vi "JTAG F-RAM Special Config.vi"() -> ()   [LabVIEW 2009]
panel:
  in  "Front Panel":T1 {"Working..." scale=0.0..1.0; "0x7FC5 - STIM ASIC REV" format="%02x"; "FRAM STIM DATA"."Data" format="%02x"; "FRAM STIM DATA"."Address" format="%04x"; "MICS_TRIMS (0x7FF0-7FFF" format="%02x"; "PWR_TRIMS (0x7FD0-7FDF" format="%02x"; "STIM_TRIMS (0x7FE0-7FEF" format="%02x"}
  # "0x7FC0 - STARTUP"
  # "0x7FC4 - SPCL TEST"
  # "0x7FC1 - STIM"
  # "0x7FC2 - PWR"
  # "0x7FC3 - MICS"
  # "BG_TRIM"
  # "PWR_TRIM0"
  # "TX RF Power"
  # "CG_TRIM"
  # "PWR_TRIM1"
  # "TxPort_TxMode"
  # "PGO_TRIM"
  # "PWR_TRIM2"
  # "TxPort_RxMode"
  # "CM_TRIM"
  # "PWR_TRIM3"
  # "RxPort_TxMode"
  # "<Reserved>"
  # "PWR_TRIM4"
  # "RxPort_RxMode"
  # "<Reserved>"
  # "PWR_TRIM5"
  # "Ant_Match1"
  # "<Reserved>"
  # "PWR_TRIM6"
  # "Ant_Match2"
  # "<Reserved>"
  # "PWR_TRIM7"
  # "MICS Channel"
  # "<Reserved>"
  # "PWR_TRIM8"
  # "TX Modulation"
  # "<Reserved>"
  # "PWR_TRIM9"
  # "<Reserved>"
  # "<Reserved>"
  # "PWR_TRIM10"
  # "<Reserved>"
  # "<Reserved>"
  # "<Reserved>"
  # "<Reserved>"
  # "<Reserved>"
  # "<Reserved>"
  # "<Reserved>"
  # "<Reserved>"
  # "<Reserved>"
  # "<Reserved>"
  # "<Reserved>"
  # "<Reserved>"
  # "mac_calselect1"
  # "<Reserved>"
  # "<Reserved>"
  # "mac_calselect2"
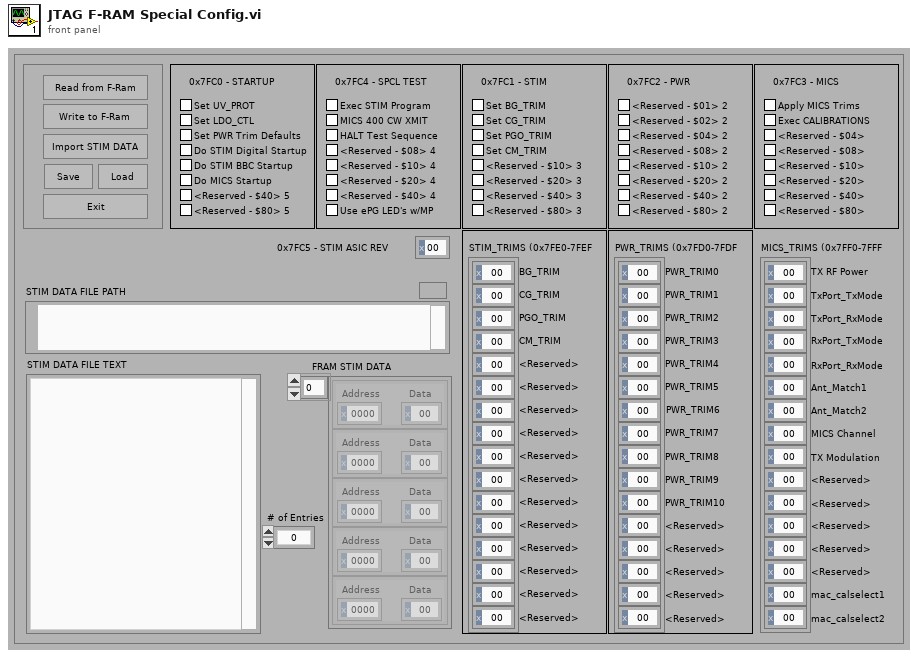
[diagram p1: front panel]
types:
  T1 = cluster{"FRAM STIM DATA":cluster{"Address":u16, "Data":u8}[], "MICS_TRIMS (0x7FF0-7FFF":u8[], "<Reserved - $80>":bool, "<Reserved - $40>":bool, "<Reserved - $20>":bool, "<Reserved - $10>":bool, "<Reserved - $08>":bool, "<Reserved - $04>":bool, "Exec CALIBRATIONS":bool, "Apply MICS Trims":bool, "PWR_TRIMS (0x7FD0-7FDF":u8[], "STIM_TRIMS (0x7FE0-7FEF":u8[], "<Reserved - $80> 2":bool, "<Reserved - $40> 2":bool, "<Reserved - $20> 2":bool, "<Reserved - $10> 2":bool, "<Reserved - $08> 2":bool, "<Reserved - $04> 2":bool, "<Reserved - $02> 2":bool, "<Reserved - $01> 2":bool, "<Reserved - $80> 3":bool, "<Reserved - $40> 3":bool, "<Reserved - $20> 3":bool, "<Reserved - $10> 3":bool, "Set CM_TRIM":bool, "Set PGO_TRIM":bool, "Set CG_TRIM":bool, "Set BG_TRIM":bool, "Use ePG LED's w/MP":bool, "<Reserved - $40> 4":bool, "<Reserved - $20> 4":bool, "<Reserved - $10> 4":bool, "<Reserved - $08> 4":bool, "HALT Test Sequence":bool, "MICS 400 CW XMIT":bool, "Exec STIM Program":bool, "<Reserved - $80> 5":bool, "<Reserved - $40> 5":bool, "Do MICS Startup":bool, "Do STIM BBC Startup":bool, "Do STIM Digital Startup":bool, "Set PWR Trim Defaults":bool, "Set LDO_CTL":bool, "Set UV_PROT":bool, "STIM DATA FILE PATH":path, "STIM DATA FILE TEXT":string, "# of Entries":u16, "User Controls":cluster{"Exit":bool, "Import Stim Prog":bool, "Write to F-Ram":bool, "Read from F-Ram":bool, "Save":bool, "Load":bool}, "0x7FC5 - STIM ASIC REV":u8, "Working...":dbl}
  T2 = cluster{"STIM PROGRAM FRAM DATA":cluster{"Address":u16, "Data":u8}[], "MICS_TRIMS (0x7FF0-7FFF":u8[], "<Reserved - $80>":bool, "<Reserved - $40>":bool, "<Reserved - $20>":bool, "<Reserved - $10>":bool, "<Reserved - $08>":bool, "<Reserved - $04>":bool, "<Reserved - $02>":bool, "<Reserved - $01>":bool, "PWR_TRIMS (0x7FD0-7FDF":u8[], "STIM_TRIMS (0x7FE0-7FEF":u8[], "<Reserved - $80> 2":bool, "<Reserved - $40> 2":bool, "<Reserved - $20> 2":bool, "<Reserved - $10> 2":bool, "<Reserved - $08> 2":bool, "<Reserved - $04> 2":bool, "<Reserved - $02> 2":bool, "Apply FRAM Trims":bool, "<Reserved - $80> 3":bool, "<Reserved - $40> 3":bool, "<Reserved - $20> 3":bool, "<Reserved - $10> 3":bool, "<Reserved - $08> 3":bool, "PGO_TRIM Valid":bool, "CG_TRIM Valid":bool, "BG_TRIM Valid":bool, "Use ePG LED's w/MP":bool, "<Reserved - $40> 4":bool, "<Reserved - $20> 4":bool, "<Reserved - $10> 4":bool, "<Reserved - $08> 4":bool, "HALT Test Sequence":bool, "MICS 400 CW Mode":bool, "Load STIM Program":bool, "<Reserved - $80> 5":bool, "<Reserved - $40> 5":bool, "Do MICS Startup":bool, "Do STIM BBC Startup":bool, "Do STIM Digital Startup":bool, "Set Pluto Trim Defaults":bool, "Set LDO_CTL":bool, "Set UV_PROT":bool, "STIM PROGRAM FILE PATH":path, "STIM PROGRAM FILE TEXT":string, "# of Entries":u16, "User Controls":cluster{"Exit":bool, "Import Stim Prog":bool, "Write to F-Ram":bool, "Read from F-Ram":bool, "Save":bool, "Load":bool}, "0x7FC5 - STIM ASIC REV":u8, "Working...":dbl}
  T3 = enum16{"Power UP", "Power DN", "Read Single", "Write Single", "Read Block", "Write Block", "Read SR", "Write SR", "Send Opcode"}
  T4 = cluster{"PWR_TRIMS (0x7FD0-7FDF[0]":u8, "PWR_TRIMS (0x7FD0-7FDF[1]":u8, "PWR_TRIMS (0x7FD0-7FDF[2]":u8, "PWR_TRIMS (0x7FD0-7FDF[3]":u8, "PWR_TRIMS (0x7FD0-7FDF[4]":u8, "PWR_TRIMS (0x7FD0-7FDF[5]":u8, "PWR_TRIMS (0x7FD0-7FDF[6]":u8, "PWR_TRIMS (0x7FD0-7FDF[7]":u8, "PWR_TRIMS (0x7FD0-7FDF[8]":u8, "PWR_TRIMS (0x7FD0-7FDF[9]":u8, "PWR_TRIMS (0x7FD0-7FDF[10]":u8, "PWR_TRIMS (0x7FD0-7FDF[11]":u8, "PWR_TRIMS (0x7FD0-7FDF[12]":u8, "PWR_TRIMS (0x7FD0-7FDF[13]":u8, "PWR_TRIMS (0x7FD0-7FDF[14]":u8, "PWR_TRIMS (0x7FD0-7FDF[15]":u8}
  T5 = cluster{"STIM_TRIMS (0x7FE0-7FEF[0]":u8, "STIM_TRIMS (0x7FE0-7FEF[1]":u8, "STIM_TRIMS (0x7FE0-7FEF[2]":u8, "STIM_TRIMS (0x7FE0-7FEF[3]":u8, "STIM_TRIMS (0x7FE0-7FEF[4]":u8, "STIM_TRIMS (0x7FE0-7FEF[5]":u8, "STIM_TRIMS (0x7FE0-7FEF[6]":u8, "STIM_TRIMS (0x7FE0-7FEF[7]":u8, "STIM_TRIMS (0x7FE0-7FEF[8]":u8, "STIM_TRIMS (0x7FE0-7FEF[9]":u8, "STIM_TRIMS (0x7FE0-7FEF[10]":u8, "STIM_TRIMS (0x7FE0-7FEF[11]":u8, "STIM_TRIMS (0x7FE0-7FEF[12]":u8, "STIM_TRIMS (0x7FE0-7FEF[13]":u8, "STIM_TRIMS (0x7FE0-7FEF[14]":u8, "STIM_TRIMS (0x7FE0-7FEF[15]":u8}
  T6 = cluster{"MICS_TRIMS (0x7FF0-7FFF[0]":u8, "MICS_TRIMS (0x7FF0-7FFF[1]":u8, "MICS_TRIMS (0x7FF0-7FFF[2]":u8, "MICS_TRIMS (0x7FF0-7FFF[3]":u8, "MICS_TRIMS (0x7FF0-7FFF[4]":u8, "MICS_TRIMS (0x7FF0-7FFF[5]":u8, "MICS_TRIMS (0x7FF0-7FFF[6]":u8, "MICS_TRIMS (0x7FF0-7FFF[7]":u8, "MICS_TRIMS (0x7FF0-7FFF[8]":u8, "MICS_TRIMS (0x7FF0-7FFF[9]":u8, "MICS_TRIMS (0x7FF0-7FFF[10]":u8, "MICS_TRIMS (0x7FF0-7FFF[11]":u8, "MICS_TRIMS (0x7FF0-7FFF[12]":u8, "MICS_TRIMS (0x7FF0-7FFF[13]":u8, "MICS_TRIMS (0x7FF0-7FFF[14]":u8, "MICS_TRIMS (0x7FF0-7FFF[15]":u8}
  T7 = cluster{"Boolean array[0]":bool, "Boolean array[1]":bool, "Boolean array[2]":bool, "Boolean array[3]":bool, "Boolean array[4]":bool, "Boolean array[5]":bool, "Boolean array[6]":bool, "Boolean array[7]":bool}
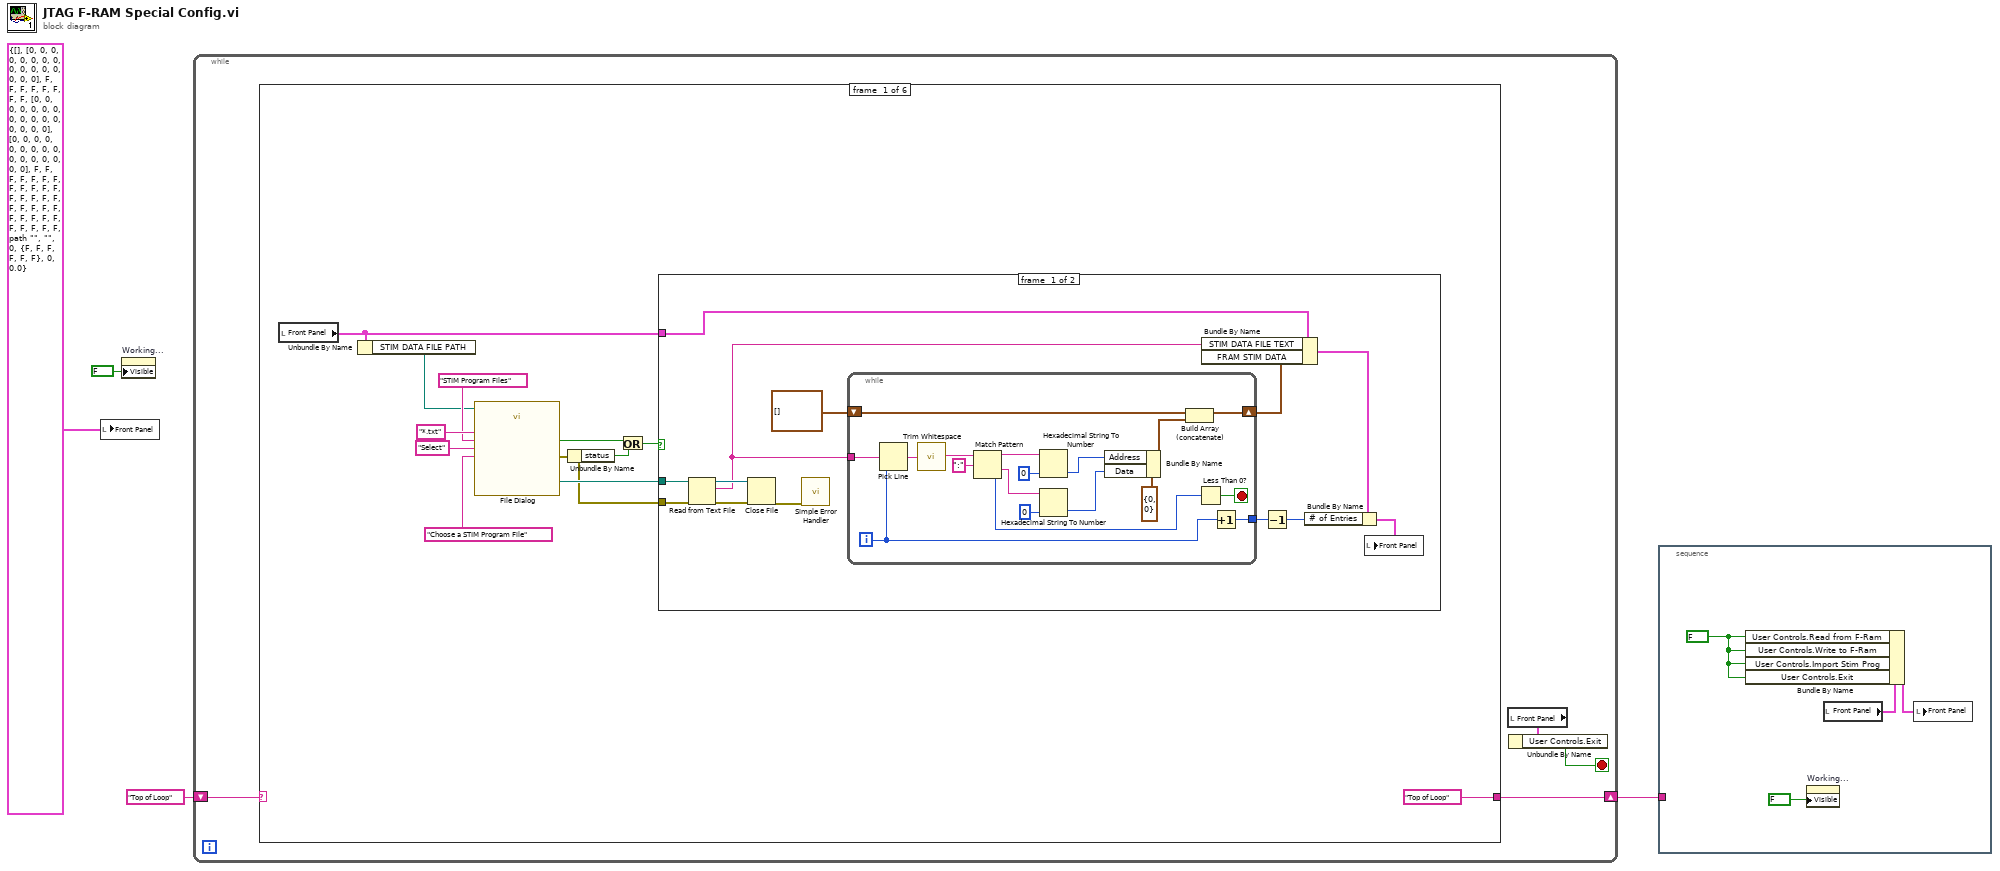
[diagram p0: block diagram]
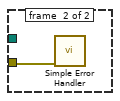
[diagram p2: hidden frame]
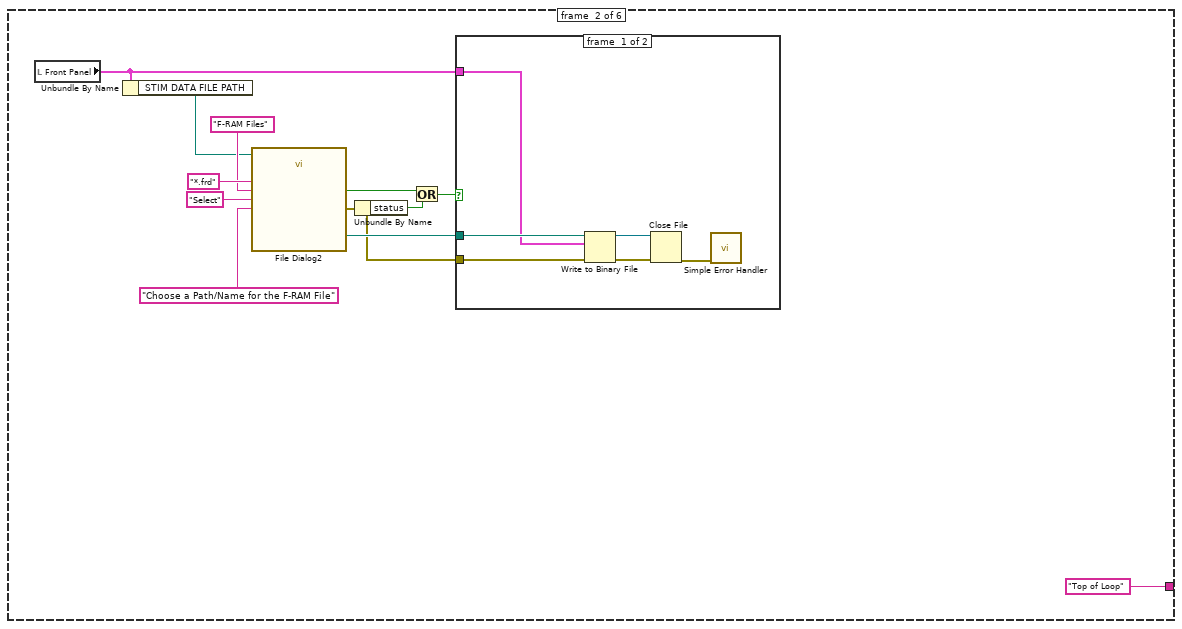
[diagram p3: hidden frame]
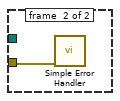
[diagram p4: hidden frame]
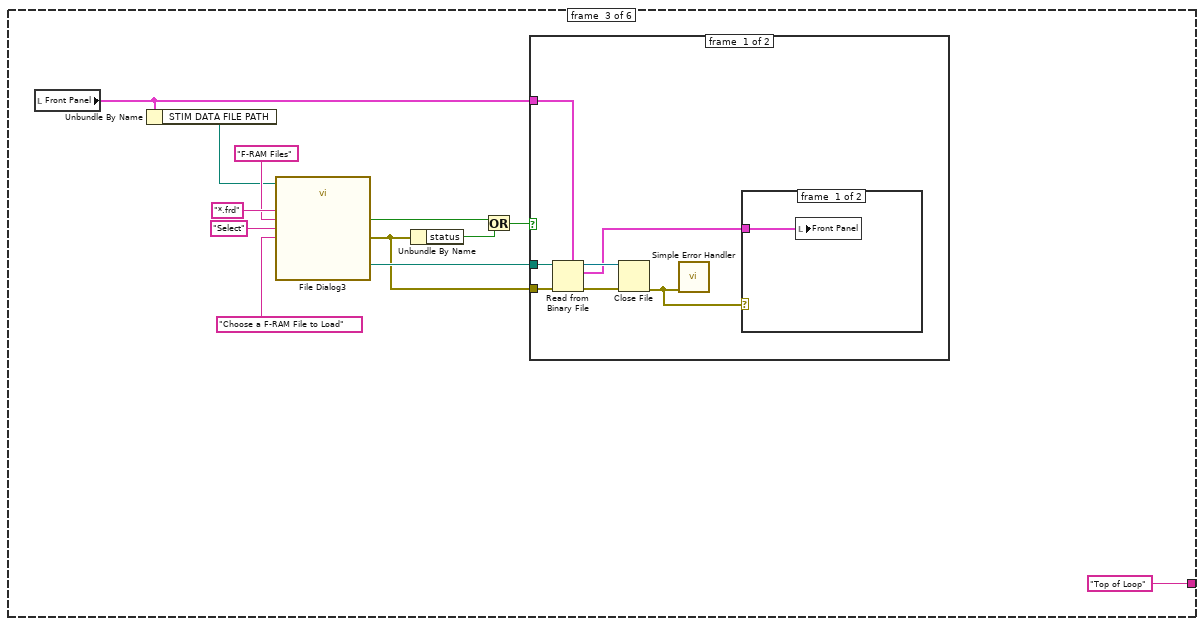
[diagram p5: hidden frame]
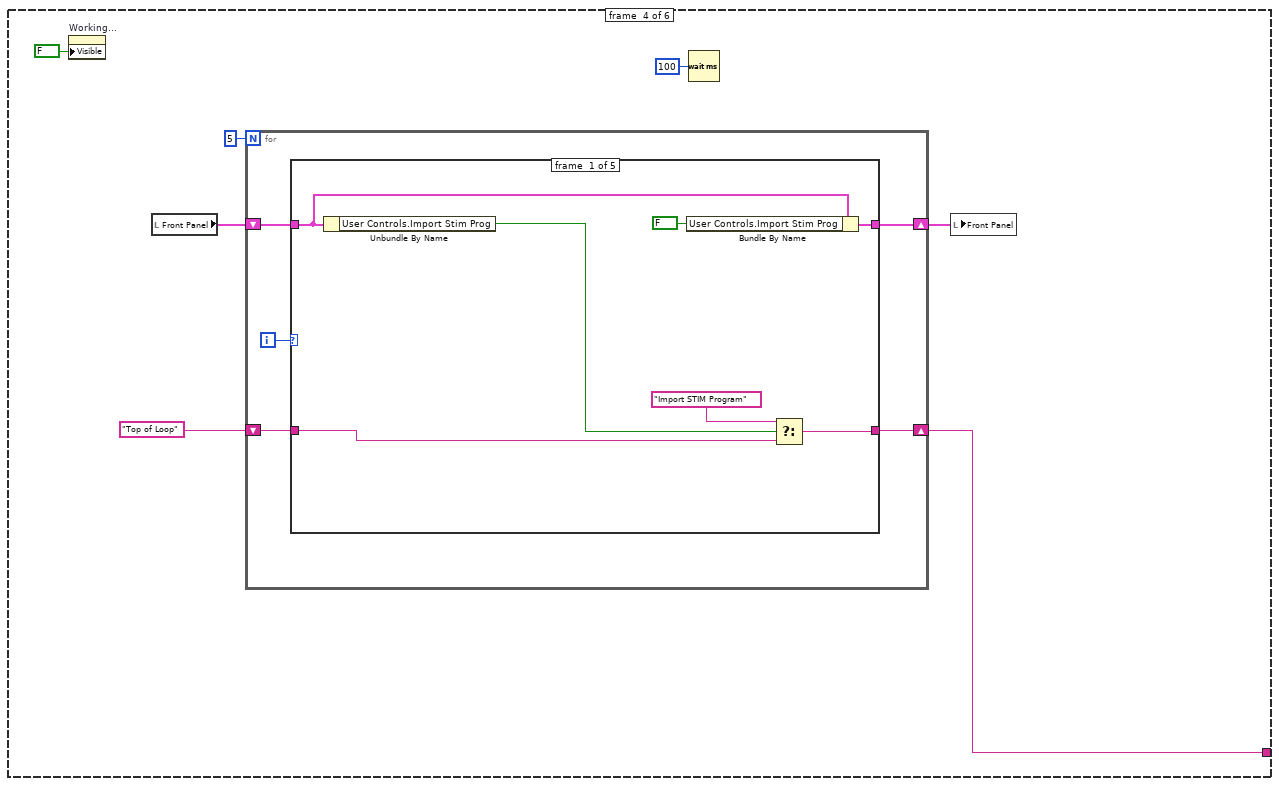
[diagram p8: hidden frame]
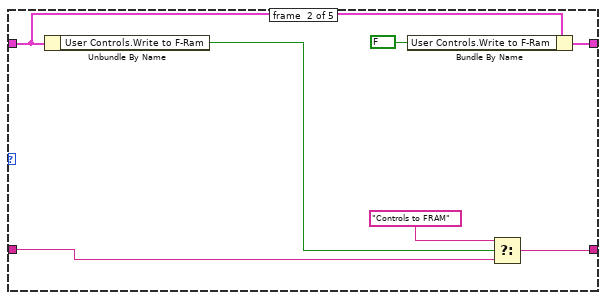
[diagram p9: hidden frame]
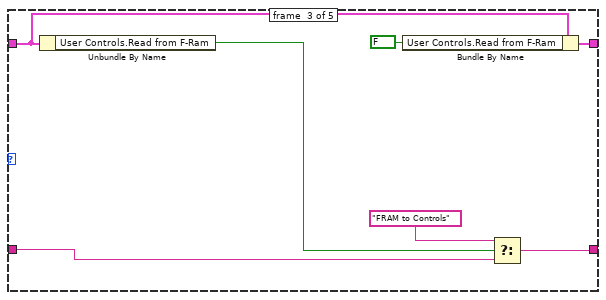
[diagram p10: hidden frame]
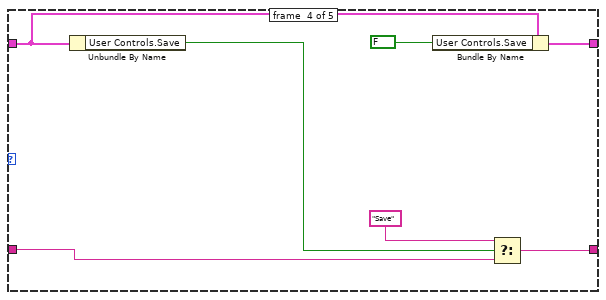
[diagram p11: hidden frame]
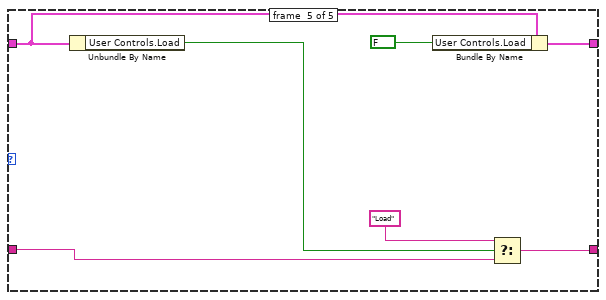
[diagram p12: hidden frame]
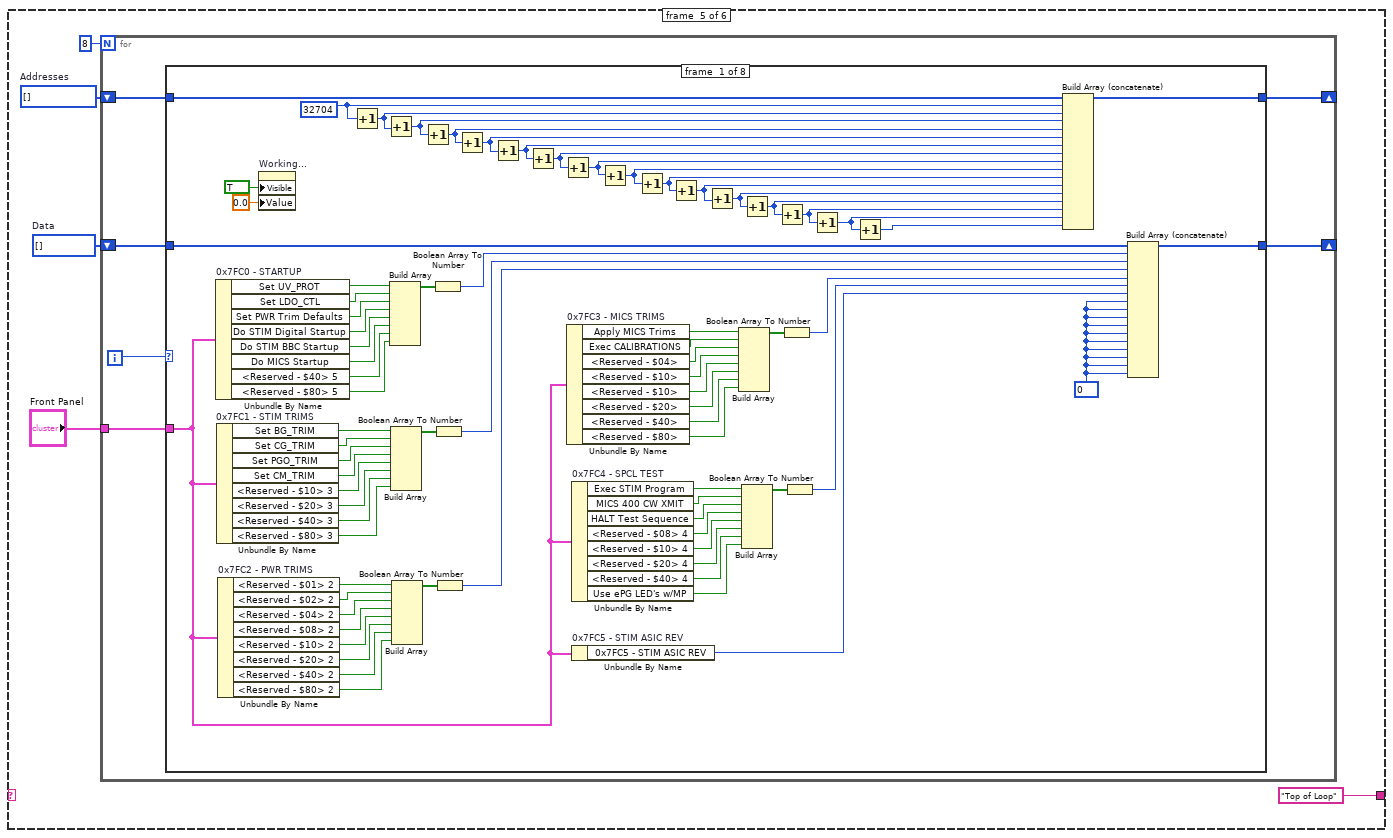
[diagram p13: hidden frame]
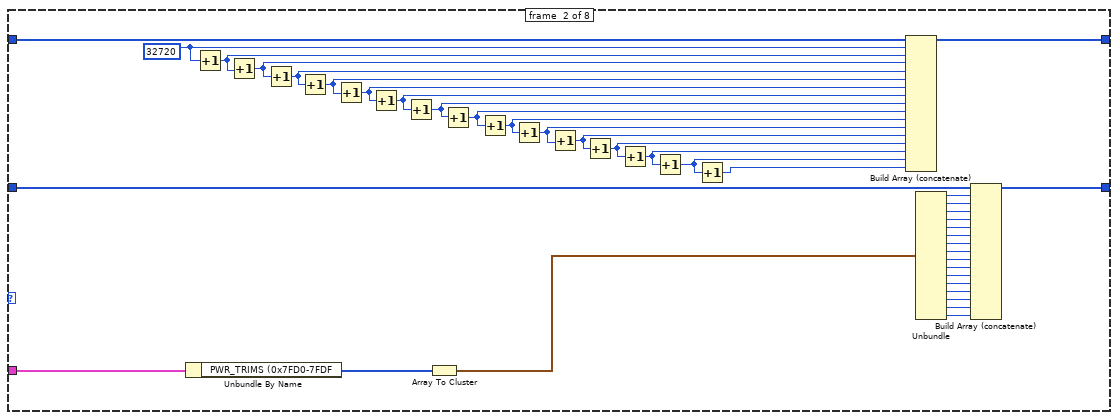
[diagram p14: hidden frame]
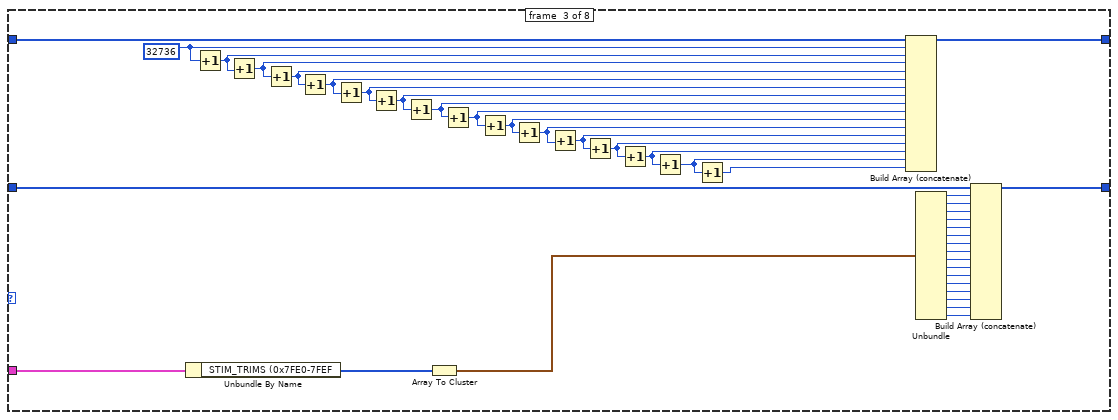
[diagram p15: hidden frame]
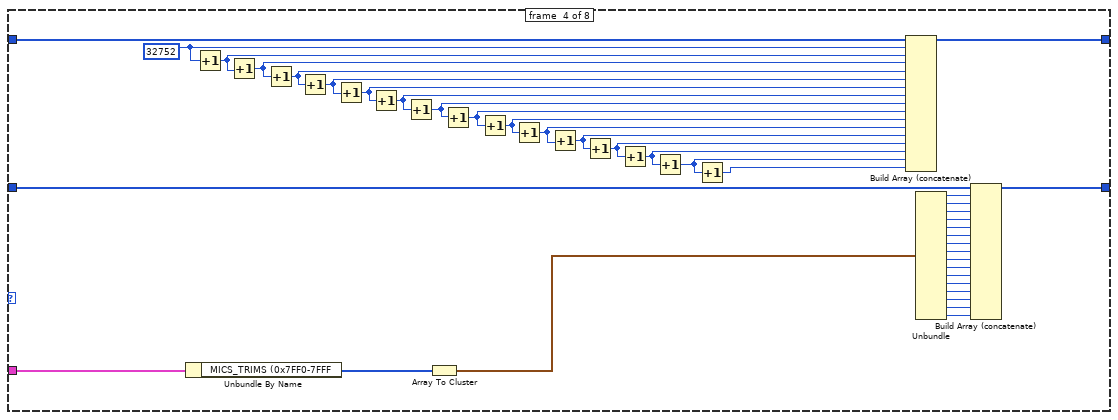
[diagram p16: hidden frame]
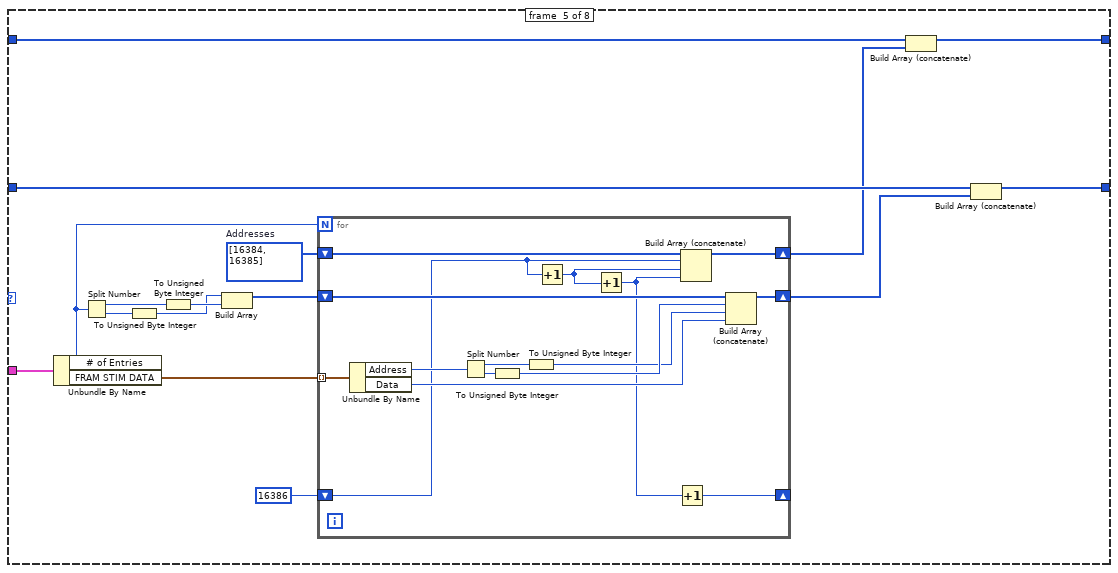
[diagram p17: hidden frame]
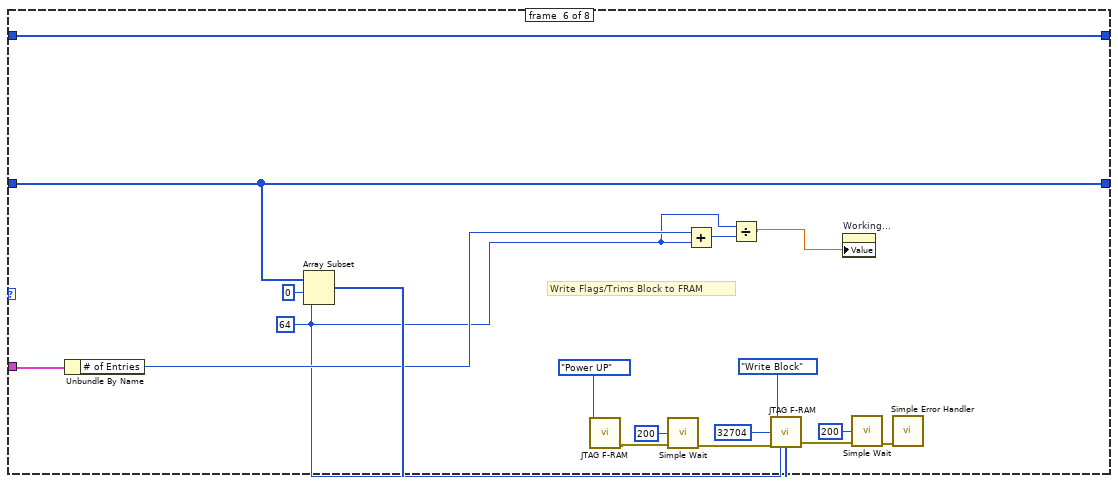
[diagram p18: hidden frame]
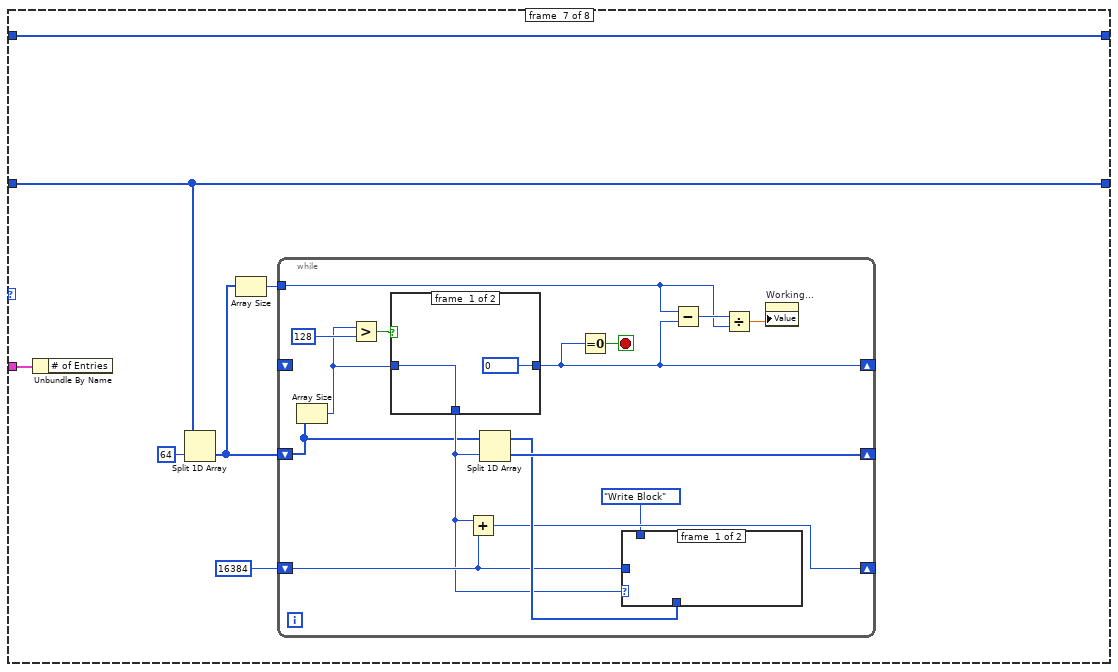
[diagram p19: hidden frame]
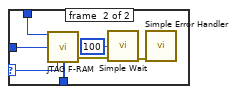
[diagram p20: hidden frame]
diagram:
  n1 = local write "Front Panel"(T2 {"STIM PROGRAM FRAM DATA"=[], "MICS_TRIMS (0x7FF0-7FFF"=[0, 0, 0, 0, 0, 0, 0, 0, 0, 0, 0, 0, 0, 0, 0, 0], "<Reserved - $80>"=FALSE, "<Reserved - $40>"=FALSE, "<Reserved - $20>"=FALSE, "<Reserved - $10>"=FALSE, "<Reserved - $08>"=FALSE, "<Reserved - $04>"=FALSE, "<Reserved - $02>"=FALSE, "<Reserved - $01>"=FALSE, "PWR_TRIMS (0x7FD0-7FDF"=[0, 0, 0, 0, 0, 0, 0, 0, 0, 0, 0, 0, 0, 0, 0, 0], "STIM_TRIMS (0x7FE0-7FEF"=[0, 0, 0, 0, 0, 0, 0, 0, 0, 0, 0, 0, 0, 0, 0, 0], "<Reserved - $80> 2"=FALSE, "<Reserved - $40> 2"=FALSE, "<Reserved - $20> 2"=FALSE, "<Reserved - $10> 2"=FALSE, "<Reserved - $08> 2"=FALSE, "<Reserved - $04> 2"=FALSE, "<Reserved - $02> 2"=FALSE, "Apply FRAM Trims"=FALSE, "<Reserved - $80> 3"=FALSE, "<Reserved - $40> 3"=FALSE, "<Reserved - $20> 3"=FALSE, "<Reserved - $10> 3"=FALSE, "<Reserved - $08> 3"=FALSE, "PGO_TRIM Valid"=FALSE, "CG_TRIM Valid"=FALSE, "BG_TRIM Valid"=FALSE, "Use ePG LED's w/MP"=FALSE, "<Reserved - $40> 4"=FALSE, "<Reserved - $20> 4"=FALSE, "<Reserved - $10> 4"=FALSE, "<Reserved - $08> 4"=FALSE, "HALT Test Sequence"=FALSE, "MICS 400 CW Mode"=FALSE, "Load STIM Program"=FALSE, "<Reserved - $80> 5"=FALSE, "<Reserved - $40> 5"=FALSE, "Do MICS Startup"=FALSE, "Do STIM BBC Startup"=FALSE, "Do STIM Digital Startup"=FALSE, "Set Pluto Trim Defaults"=FALSE, "Set LDO_CTL"=FALSE, "Set UV_PROT"=FALSE, "STIM PROGRAM FILE PATH"=path "", "STIM PROGRAM FILE TEXT"="", "# of Entries"=0, "User Controls"={"Exit"=FALSE, "Import Stim Prog"=FALSE, "Write to F-Ram"=FALSE, "Read from F-Ram"=FALSE, "Save"=FALSE, "Load"=FALSE}, "0x7FC5 - STIM ASIC REV"=0, "Working..."=0.0} ("Front Panel")) -> ()
  n2 = property on="Working..." class="Slide (strict)"("Visible"=FALSE) -> ()  [unwired: 2 in, 2 out]
  n3 = while {
    shift-right: [w5] -> w3
    shift-left: "Top of Loop" -> [w8]
    stop <- w6 stop-if-true
    n4 = case shown="\"Controls to FRAM\"" w8 {
      tunnel: ["Top of Loop" "Top of Loop" "Top of Loop" w96 "Top of Loop" "Top of Loop"] -> w5
      frame #0 {
        n5 = local read "Front Panel"() -> (w10:T1)
        n6 = Unbundle By Name(w10) -> ("STIM DATA FILE PATH"=w9:path)
        n7 = call "File Dialog"("start path"=w9, "prompt"="Choose a STIM Program File", "button label"="Select", "pattern (all files)"="*.txt", "pattern label"="STIM Program Files") -> ("selected path"=w13:path, "cancelled"=w15:bool, "error out"=w12:errorcluster)  [unwired: 7 in, 1 out]
        n8 = Unbundle By Name(w12) -> ("status"=w14:bool)
        n9 = Or(x=w15, y=w14) -> (x .or. y?=w16:bool)
        n10 = case shown="False" w16 {
          tunnel: w13 -> [w33 _]
          tunnel: w12 -> [w28 w52]
          tunnel: w10 -> [w22 _]
          frame #0 {
            n11 = Read from Text File(file (use dialog)=w33, error in=w28) -> (refnum out=w32:refnum<file>, text=w21:string, error out=w29:errorcluster)  [unwired: 2 in, 1 out]
            n12 = Close File(refnum=w32, error in=w29) -> (error out=w30:errorcluster)  [unwired: 1 out]
            n13 = call <vilib>:"Simple Error Handler.vi"("error in (no error)"=w30) -> ()  [unwired: 4 in, 5 out]
            n14 = while {
              tunnel: w21 -> [w50]
              shift-right: [w36] -> w31
              shift-left: cluster{"Address":u16, "Data":u8}[] [] ("STIM PROGRAM FRAM DATA") -> [w35]
              tunnel: [w51] -> w25
              i -> [w49]
              stop <- w41 stop-if-true
              n15 = Pick Line(multi-line string=w50, line index=w49) -> (output string=w48:string)  [unwired: 1 in]
              n16 = call <vilib>:"Trim Whitespace.vi"("string"=w48) -> ("trimmed string"=w47:string)  [unwired: 1 in]
              n17 = Match Pattern(string=w47, regular expression=":") -> (before substring=w44:string, after substring=w42:string, offset past match=w40:i32)  [unwired: 1 in, 1 out]
              n18 = Hexadecimal String To Number(string=w44, default (0uL)=u16 0) -> (number=w37:u16)  [unwired: 1 in, 1 out]
              n19 = Hexadecimal String To Number(string=w42, default (0uL)=u8 0) -> (number=w38:u8)  [unwired: 1 in, 1 out]
              n20 = Bundle By Name(cluster=cluster{"Address":u16, "Data":u8} {"Address"=0, "Data"=0} ("Cluster"), "Address"=w37, "Data"=w38) -> (w34:cluster{"Address":u16, "Data":u8})
              n21 = Build Array (concatenate)(w35, w34) -> (w36:cluster{"Address":u16, "Data":u8}[])
              n22 = Less Than 0?(x=w40) -> (x < 0?=w41:bool)
              n23 = Increment(x=w49) -> (x+1=w51:i32)
            }
            n24 = Bundle By Name(cluster=w22, "STIM DATA FILE TEXT"=w21, "FRAM STIM DATA"=w31) -> (w27:T1)
            n25 = Decrement(x=w25) -> (x-1=w24:i32)
            n26 = Bundle By Name(cluster=w27, "# of Entries"=w24) -> (w26:T1)
            n27 = local write "Front Panel"(w26) -> ()
          }
          frame #1 {
            n28 = call <vilib>:"Simple Error Handler.vi"("error in (no error)"=w52) -> ()  [unwired: 4 in, 5 out]
          }
        }
      }
      frame #1 {
        n29 = local read "Front Panel"() -> (w54:T1)
        n30 = Unbundle By Name(w54) -> ("STIM DATA FILE PATH"=w53:path)
        n31 = call "File Dialog2"("start path"=w53, "prompt"="Choose a Path/Name for the F-RAM File", "button label"="Select", "pattern (all files)"="*.frd", "pattern label"="F-RAM Files") -> ("selected path"=w57:path, "cancelled"=w59:bool, "error out"=w56:errorcluster)  [unwired: 7 in, 1 out]
        n32 = Unbundle By Name(w56) -> ("status"=w58:bool)
        n33 = Or(x=w59, y=w58) -> (x .or. y?=w60:bool)
        n34 = case shown="False" w60 {
          tunnel: w57 -> [w70 _]
          tunnel: w56 -> [w66 w71]
          tunnel: w54 -> [w65 _]
          frame #0 {
            n35 = Write to Binary File(file (use dialog)=w70, data=w65, error in=w66) -> (refnum out=w69:refnum<file>, error out=w67:errorcluster)  [unwired: 3 in, 1 out]
            n36 = Close File(refnum=w69, error in=w67) -> (error out=w68:errorcluster)  [unwired: 1 out]
            n37 = call <vilib>:"Simple Error Handler.vi"("error in (no error)"=w68) -> ()  [unwired: 4 in, 5 out]
          }
          frame #1 {
            n38 = call <vilib>:"Simple Error Handler.vi"("error in (no error)"=w71) -> ()  [unwired: 4 in, 5 out]
          }
        }
      }
      frame #2 {
        n39 = local read "Front Panel"() -> (w73:T1)
        n40 = Unbundle By Name(w73) -> ("STIM DATA FILE PATH"=w72:path)
        n41 = call "File Dialog3"("start path"=w72, "prompt"="Choose a F-RAM File to Load", "button label"="Select", "pattern (all files)"="*.frd", "pattern label"="F-RAM Files") -> ("selected path"=w76:path, "cancelled"=w78:bool, "error out"=w75:errorcluster)  [unwired: 7 in, 1 out]
        n42 = Unbundle By Name(w75) -> ("status"=w77:bool)
        n43 = Or(x=w78, y=w77) -> (x .or. y?=w79:bool)
        n44 = case shown="False" w79 {
          tunnel: w76 -> [w90 _]
          tunnel: w75 -> [w87 w92]
          tunnel: w73 -> [w85 _]
          frame #0 {
            n45 = Read from Binary File(5:w85, 8:w87, 11:w90) -> (0:w88:errorcluster, 2:w84:T1, 3:w89:refnum<file>)  [unwired: 3 in, 1 out]
            n46 = Close File(refnum=w89, error in=w88) -> (error out=w86:errorcluster)  [unwired: 1 out]
            n47 = call <vilib>:"Simple Error Handler.vi"("error in (no error)"=w86) -> ()  [unwired: 4 in, 5 out]
            n48 = case shown="No Error" w86 {
              tunnel: w84 -> [w91 _]
              frame #0 {
                n49 = local write "Front Panel"(w91) -> ()
              }
              frame #1 {
              }
            }
          }
          frame #1 {
            n50 = call <vilib>:"Simple Error Handler.vi"("error in (no error)"=w92) -> ()  [unwired: 4 in, 5 out]
          }
        }
      }
      frame #3 {
        n51 = property on="Working..." class="Slide (strict)"("Visible"=FALSE) -> ()  [unwired: 2 in, 2 out]
        n52 = local read "Front Panel"() -> (w99:T1)
        n53 = for {
          N: 5 -> [_]
          shift-right: [w104] -> w98
          shift-left: w99 -> [w103]
          shift-right: [w101] -> w96
          shift-left: "Top of Loop" -> [w100]
          i -> [w102]
          n54 = case shown="4" w102 {
            tunnel: [w111 w118 w125 w132 w139] -> w104
            tunnel: w103 -> [w110 w117 w124 w131 w138]
            tunnel: [w108 w115 w122 w129 w136] -> w101
            tunnel: w100 -> [w105 w112 w119 w126 w133]
            frame #0 {
              n55 = Unbundle By Name(w110) -> ("User Controls.Import Stim Prog"=w107:bool)
              n56 = Bundle By Name(cluster=w110, "User Controls.Import Stim Prog"=FALSE) -> (w111:T1)
              n57 = Select(t="Import STIM Program", s=w107, f=w105) -> (s? t:f=w108:string)
            }
            frame #1 {
              n58 = Unbundle By Name(w117) -> ("User Controls.Write to F-Ram"=w114:bool)
              n59 = Bundle By Name(cluster=w117, "User Controls.Write to F-Ram"=FALSE ("User Controls.Import Stim Prog")) -> (w118:T1)
              n60 = Select(t="Controls to FRAM", s=w114, f=w112) -> (s? t:f=w115:string)
            }
            frame #2 {
              n61 = Unbundle By Name(w124) -> ("User Controls.Read from F-Ram"=w121:bool)
              n62 = Bundle By Name(cluster=w124, "User Controls.Read from F-Ram"=FALSE ("User Controls.Import Stim Prog")) -> (w125:T1)
              n63 = Select(t="FRAM to Controls", s=w121, f=w119) -> (s? t:f=w122:string)
            }
            frame #3 {
              n64 = Unbundle By Name(w131) -> ("User Controls.Save"=w128:bool)
              n65 = Bundle By Name(cluster=w131, "User Controls.Save"=FALSE ("User Controls.Import Stim Prog")) -> (w132:T1)
              n66 = Select(t="Save", s=w128, f=w126) -> (s? t:f=w129:string)
            }
            frame #4 {
              n67 = Unbundle By Name(w138) -> ("User Controls.Load"=w135:bool)
              n68 = Bundle By Name(cluster=w138, "User Controls.Load"=FALSE ("User Controls.Import Stim Prog")) -> (w139:T1)
              n69 = Select(t="Load", s=w135, f=w133) -> (s? t:f=w136:string)
            }
          }
        }
        n70 = Wait (ms)(milliseconds to wait=u32 100) -> ()  [unwired: 1 out]
        n71 = local write "Front Panel"(w98) -> ()
      }
      frame #4 {
        w142 = u8[] []  # Data
        w143 = u16[] []  # Addresses
        n72 = for {
          N: 8 -> [_]
          tunnel: "Front Panel" -> [w147]
          shift-right: [w145] -> _
          shift-left: w143 -> [w150]
          shift-right: [w146] -> _
          shift-left: w142 -> [w149]
          i -> [w148]
          n73 = case shown="0, Default" w148 {
            tunnel: w150 -> [w224 w263 w302 w341 w357 w391 w398 w428]
            tunnel: w149 -> [w222 w261 w300 w339 w355 w390 w396 w429]
            tunnel: w147 -> [w154 w260 w299 w338 w354 w378 w397 _]
            tunnel: [w223 w262 w301 w340 w356 w390 w396 w429] -> w146
            tunnel: [w225 w264 w303 w342 w358 w391 w398 w428] -> w145
            frame #0 {
              w171 = u16 32704
              w157 = u8 0
              n74 = Unbundle By Name "0x7FC0 - STARTUP"(w154) -> ("Set UV_PROT"=w200:bool, "Set LDO_CTL"=w199:bool, "Set PWR Trim Defaults"=w198:bool, "Do STIM Digital Startup"=w197:bool, "Do STIM BBC Startup"=w196:bool, "Do MICS Startup"=w195:bool, "<Reserved - $40> 5"=w194:bool, "<Reserved - $80> 5"=w193:bool)
              n75 = Unbundle By Name "0x7FC1 - STIM TRIMS"(w154) -> ("Set BG_TRIM"=w208:bool, "Set CG_TRIM"=w207:bool, "Set PGO_TRIM"=w206:bool, "Set CM_TRIM"=w205:bool, "<Reserved - $10> 3"=w204:bool, "<Reserved - $20> 3"=w203:bool, "<Reserved - $40> 3"=w202:bool, "<Reserved - $80> 3"=w201:bool)
              n76 = Unbundle By Name "0x7FC2 - PWR TRIMS"(w154) -> ("<Reserved - $01> 2"=w216:bool, "<Reserved - $02> 2"=w215:bool, "<Reserved - $04> 2"=w214:bool, "<Reserved - $08> 2"=w213:bool, "<Reserved - $10> 2"=w212:bool, "<Reserved - $20> 2"=w211:bool, "<Reserved - $40> 2"=w210:bool, "<Reserved - $80> 2"=w209:bool)
              n77 = property on="Working..." class="Slide (strict)"("Visible"=TRUE, "Value"=0.0) -> ()  [unwired: 2 in, 2 out]
              n78 = Increment(x=w171) -> (x+1=w170:u16)
              n79 = Increment(x=w170) -> (x+1=w169:u16)
              n80 = Build Array(w200, w199, w198, w197, w196, w195, w194, w193) -> (w219:bool[])
              n81 = Build Array(w208, w207, w206, w205, w204, w203, w202, w201) -> (w218:bool[])
              n82 = Build Array(w216, w215, w214, w213, w212, w211, w210, w209) -> (w217:bool[])
              n83 = Increment(x=w169) -> (x+1=w168:u16)
              n84 = Boolean Array To Number(Boolean array=w219) -> (number=w176:u8)
              n85 = Boolean Array To Number(Boolean array=w218) -> (number=w175:u8)
              n86 = Boolean Array To Number(Boolean array=w217) -> (number=w174:u8)
              n87 = Increment(x=w168) -> (x+1=w167:u16)
              n88 = Increment(x=w167) -> (x+1=w166:u16)
              n89 = Increment(x=w166) -> (x+1=w165:u16)
              n90 = Increment(x=w165) -> (x+1=w164:u16)
              n91 = Unbundle By Name "0x7FC3 - MICS TRIMS"(w154) -> ("Apply MICS Trims"=w192:bool, "Exec CALIBRATIONS"=w191:bool, "<Reserved - $04>"=w190:bool, "<Reserved - $10>"=w189:bool, "<Reserved - $10>"=w188:bool, "<Reserved - $20>"=w187:bool, "<Reserved - $40>"=w186:bool, "<Reserved - $80>"=w185:bool)
              n92 = Unbundle By Name "0x7FC4 - SPCL TEST"(w154) -> ("Exec STIM Program"=w184:bool, "MICS 400 CW XMIT"=w183:bool, "HALT Test Sequence"=w182:bool, "<Reserved - $08> 4"=w181:bool, "<Reserved - $10> 4"=w180:bool, "<Reserved - $20> 4"=w179:bool, "<Reserved - $40> 4"=w178:bool, "Use ePG LED's w/MP"=w177:bool)
              n93 = Unbundle By Name "0x7FC5 - STIM ASIC REV"(w154) -> ("0x7FC5 - STIM ASIC REV"=w153:u8)
              n94 = Increment(x=w164) -> (x+1=w163:u16)
              n95 = Increment(x=w163) -> (x+1=w162:u16)
              n96 = Increment(x=w162) -> (x+1=w161:u16)
              n97 = Increment(x=w161) -> (x+1=w160:u16)
              n98 = Build Array(w192, w191, w190, w189, w188, w187, w186, w185) -> (w221:bool[])
              n99 = Increment(x=w160) -> (x+1=w159:u16)
              n100 = Build Array(w184, w183, w182, w181, w180, w179, w178, w177) -> (w220:bool[])
              n101 = Increment(x=w159) -> (x+1=w158:u16)
              n102 = Boolean Array To Number(Boolean array=w221) -> (number=w173:u8)
              n103 = Boolean Array To Number(Boolean array=w220) -> (number=w172:u8)
              n104 = Increment(x=w158) -> (x+1=w156:u16)
              n105 = Increment(x=w156) -> (x+1=w155:u16)
              n106 = Build Array (concatenate)(w224, w171, w170, w169, w168, w167, w166, w165, w164, w163, w162, w161, w160, w159, w158, w156, w155) -> (w225:u16[])
              n107 = Build Array (concatenate)(w222, w176, w175, w174, w173, w172, w153, w157, w157, w157, w157, w157, w157, w157, w157, w157, w157) -> (w223:u8[])
            }
            frame #1 {
              w259 = u16 32720
              n108 = Unbundle By Name(w260) -> ("PWR_TRIMS (0x7FD0-7FDF"=w245:u8[])
              n109 = Increment(x=w259) -> (x+1=w258:u16)
              n110 = Increment(x=w258) -> (x+1=w257:u16)
              n111 = Increment(x=w257) -> (x+1=w256:u16)
              n112 = Increment(x=w256) -> (x+1=w255:u16)
              n113 = Increment(x=w255) -> (x+1=w254:u16)
              n114 = Increment(x=w254) -> (x+1=w253:u16)
              n115 = Increment(x=w253) -> (x+1=w252:u16)
              n116 = Array To Cluster(array=w245) -> (cluster=w244:T4)
              n117 = Increment(x=w252) -> (x+1=w251:u16)
              n118 = Increment(x=w251) -> (x+1=w250:u16)
              n119 = Increment(x=w250) -> (x+1=w249:u16)
              n120 = Increment(x=w249) -> (x+1=w248:u16)
              n121 = Increment(x=w248) -> (x+1=w247:u16)
              n122 = Increment(x=w247) -> (x+1=w246:u16)
              n123 = Increment(x=w246) -> (x+1=w243:u16)
              n124 = Increment(x=w243) -> (x+1=w242:u16)
              n125 = Build Array (concatenate)(w263, w259, w258, w257, w256, w255, w254, w253, w252, w251, w250, w249, w248, w247, w246, w243, w242) -> (w264:u16[])
              n126 = Unbundle(w244) -> ("PWR_TRIMS (0x7FD0-7FDF[0]"=w226:u8, "PWR_TRIMS (0x7FD0-7FDF[1]"=w227:u8, "PWR_TRIMS (0x7FD0-7FDF[2]"=w228:u8, "PWR_TRIMS (0x7FD0-7FDF[3]"=w229:u8, "PWR_TRIMS (0x7FD0-7FDF[4]"=w230:u8, "PWR_TRIMS (0x7FD0-7FDF[5]"=w231:u8, "PWR_TRIMS (0x7FD0-7FDF[6]"=w232:u8, "PWR_TRIMS (0x7FD0-7FDF[7]"=w233:u8, "PWR_TRIMS (0x7FD0-7FDF[8]"=w234:u8, "PWR_TRIMS (0x7FD0-7FDF[9]"=w235:u8, "PWR_TRIMS (0x7FD0-7FDF[10]"=w236:u8, "PWR_TRIMS (0x7FD0-7FDF[11]"=w237:u8, "PWR_TRIMS (0x7FD0-7FDF[12]"=w238:u8, "PWR_TRIMS (0x7FD0-7FDF[13]"=w239:u8, "PWR_TRIMS (0x7FD0-7FDF[14]"=w240:u8, "PWR_TRIMS (0x7FD0-7FDF[15]"=w241:u8)
              n127 = Build Array (concatenate)(w261, w226, w227, w228, w229, w230, w231, w232, w233, w234, w235, w236, w237, w238, w239, w240, w241) -> (w262:u8[])
            }
            frame #2 {
              w298 = u16 32736
              n128 = Unbundle By Name(w299) -> ("STIM_TRIMS (0x7FE0-7FEF"=w284:u8[])
              n129 = Increment(x=w298) -> (x+1=w297:u16)
              n130 = Increment(x=w297) -> (x+1=w296:u16)
              n131 = Increment(x=w296) -> (x+1=w295:u16)
              n132 = Increment(x=w295) -> (x+1=w294:u16)
              n133 = Increment(x=w294) -> (x+1=w293:u16)
              n134 = Increment(x=w293) -> (x+1=w292:u16)
              n135 = Increment(x=w292) -> (x+1=w291:u16)
              n136 = Array To Cluster(array=w284) -> (cluster=w283:T5)
              n137 = Increment(x=w291) -> (x+1=w290:u16)
              n138 = Increment(x=w290) -> (x+1=w289:u16)
              n139 = Increment(x=w289) -> (x+1=w288:u16)
              n140 = Increment(x=w288) -> (x+1=w287:u16)
              n141 = Increment(x=w287) -> (x+1=w286:u16)
              n142 = Increment(x=w286) -> (x+1=w285:u16)
              n143 = Increment(x=w285) -> (x+1=w282:u16)
              n144 = Increment(x=w282) -> (x+1=w281:u16)
              n145 = Build Array (concatenate)(w302, w298, w297, w296, w295, w294, w293, w292, w291, w290, w289, w288, w287, w286, w285, w282, w281) -> (w303:u16[])
              n146 = Unbundle(w283) -> ("STIM_TRIMS (0x7FE0-7FEF[0]"=w265:u8, "STIM_TRIMS (0x7FE0-7FEF[1]"=w266:u8, "STIM_TRIMS (0x7FE0-7FEF[2]"=w267:u8, "STIM_TRIMS (0x7FE0-7FEF[3]"=w268:u8, "STIM_TRIMS (0x7FE0-7FEF[4]"=w269:u8, "STIM_TRIMS (0x7FE0-7FEF[5]"=w270:u8, "STIM_TRIMS (0x7FE0-7FEF[6]"=w271:u8, "STIM_TRIMS (0x7FE0-7FEF[7]"=w272:u8, "STIM_TRIMS (0x7FE0-7FEF[8]"=w273:u8, "STIM_TRIMS (0x7FE0-7FEF[9]"=w274:u8, "STIM_TRIMS (0x7FE0-7FEF[10]"=w275:u8, "STIM_TRIMS (0x7FE0-7FEF[11]"=w276:u8, "STIM_TRIMS (0x7FE0-7FEF[12]"=w277:u8, "STIM_TRIMS (0x7FE0-7FEF[13]"=w278:u8, "STIM_TRIMS (0x7FE0-7FEF[14]"=w279:u8, "STIM_TRIMS (0x7FE0-7FEF[15]"=w280:u8)
              n147 = Build Array (concatenate)(w300, w265, w266, w267, w268, w269, w270, w271, w272, w273, w274, w275, w276, w277, w278, w279, w280) -> (w301:u8[])
            }
            frame #3 {
              w337 = u16 32752
              n148 = Unbundle By Name(w338) -> ("MICS_TRIMS (0x7FF0-7FFF"=w323:u8[])
              n149 = Increment(x=w337) -> (x+1=w336:u16)
              n150 = Increment(x=w336) -> (x+1=w335:u16)
              n151 = Increment(x=w335) -> (x+1=w334:u16)
              n152 = Increment(x=w334) -> (x+1=w333:u16)
              n153 = Increment(x=w333) -> (x+1=w332:u16)
              n154 = Increment(x=w332) -> (x+1=w331:u16)
              n155 = Increment(x=w331) -> (x+1=w330:u16)
              n156 = Array To Cluster(array=w323) -> (cluster=w322:T6)
              n157 = Increment(x=w330) -> (x+1=w329:u16)
              n158 = Increment(x=w329) -> (x+1=w328:u16)
              n159 = Increment(x=w328) -> (x+1=w327:u16)
              n160 = Increment(x=w327) -> (x+1=w326:u16)
              n161 = Increment(x=w326) -> (x+1=w325:u16)
              n162 = Increment(x=w325) -> (x+1=w324:u16)
              n163 = Increment(x=w324) -> (x+1=w321:u16)
              n164 = Increment(x=w321) -> (x+1=w320:u16)
              n165 = Build Array (concatenate)(w341, w337, w336, w335, w334, w333, w332, w331, w330, w329, w328, w327, w326, w325, w324, w321, w320) -> (w342:u16[])
              n166 = Unbundle(w322) -> ("MICS_TRIMS (0x7FF0-7FFF[0]"=w304:u8, "MICS_TRIMS (0x7FF0-7FFF[1]"=w305:u8, "MICS_TRIMS (0x7FF0-7FFF[2]"=w306:u8, "MICS_TRIMS (0x7FF0-7FFF[3]"=w307:u8, "MICS_TRIMS (0x7FF0-7FFF[4]"=w308:u8, "MICS_TRIMS (0x7FF0-7FFF[5]"=w309:u8, "MICS_TRIMS (0x7FF0-7FFF[6]"=w310:u8, "MICS_TRIMS (0x7FF0-7FFF[7]"=w311:u8, "MICS_TRIMS (0x7FF0-7FFF[8]"=w312:u8, "MICS_TRIMS (0x7FF0-7FFF[9]"=w313:u8, "MICS_TRIMS (0x7FF0-7FFF[10]"=w314:u8, "MICS_TRIMS (0x7FF0-7FFF[11]"=w315:u8, "MICS_TRIMS (0x7FF0-7FFF[12]"=w316:u8, "MICS_TRIMS (0x7FF0-7FFF[13]"=w317:u8, "MICS_TRIMS (0x7FF0-7FFF[14]"=w318:u8, "MICS_TRIMS (0x7FF0-7FFF[15]"=w319:u8)
              n167 = Build Array (concatenate)(w339, w304, w305, w306, w307, w308, w309, w310, w311, w312, w313, w314, w315, w316, w317, w318, w319) -> (w340:u8[])
            }
            frame #4 {
              w352 = u16[] [16384, 16385]  # Addresses
              n168 = Unbundle By Name(w354) -> ("# of Entries"=w347:u16, "FRAM STIM DATA"=w349:cluster{"Address":u16, "Data":u8}[])
              n169 = Split Number(x=w347) -> (hi(x)=w345:u8, lo(x)=w346:u8)
              n170 = To Unsigned Byte Integer(number=w346) -> (unsigned 8bit integer=w343:u8)
              n171 = To Unsigned Byte Integer(number=w345) -> (unsigned 8bit integer=w344:u8)
              n172 = Build Array(w343, w344) -> (w348:u8[])
              n173 = for {
                N: w347 -> [_]
                shift-right: [w359] -> _
                shift-left: u16 16386 -> [w362]
                shift-right: [w369] -> w350
                shift-left: w348 -> [w372]
                shift-right: [w370] -> w351
                shift-left: w352 -> [w371]
                tunnel: w349 -> [w373] mode=indexing
                n174 = Unbundle By Name(w373) -> ("Address"=w363:u16, "Data"=w364:u8)
                n175 = Split Number(x=w363) -> (hi(x)=w367:u8, lo(x)=w368:u8)
                n176 = To Unsigned Byte Integer(number=w368) -> (unsigned 8bit integer=w366:u8)
                n177 = To Unsigned Byte Integer(number=w367) -> (unsigned 8bit integer=w365:u8)
                n178 = Increment(x=w362) -> (x+1=w361:u16)
                n179 = Increment(x=w361) -> (x+1=w360:u16)
                n180 = Increment(x=w360) -> (x+1=w359:u16)
                n181 = Build Array (concatenate)(w371, w362, w361, w360) -> (w370:u16[])
                n182 = Build Array (concatenate)(w372, w366, w365, w364) -> (w369:u8[])
              }
              n183 = Build Array (concatenate)(w357, w351) -> (w358:u16[])
              n184 = Build Array (concatenate)(w355, w350) -> (w356:u8[])
            }
            frame #5 {
              w375 = u16 64 ("length")
              # "Write Flags/Trims Block to FRAM"
              n185 = Unbundle By Name(w378) -> ("# of Entries"=w377:u16)
              n186 = Array Subset(array=w390, index=0, length=w375) -> (w388:u8[])
              n187 = call "JTAG F-RAM.vi"("Function"=T3."Power UP") -> ("error out"=w384:errorcluster)  [unwired: 12 in, 2 out]
              n188 = call "Simple Wait.vi"("mS"=u32 200, "error in"=w384) -> ("error out"=w382:errorcluster)  [unwired: 12 in, 1 out]
              n189 = Add(x=w377, y=w375) -> (x+y=w376:u16)
              n190 = Divide(x=w375, y=w376) -> (x/y=w374:dbl)
              n191 = call "JTAG F-RAM.vi"("Function"=T3."Write Block", "Address"=u16 32704, "error in (no error)"=w382, "Blocksize"=w375, "Block Write Data"=w388) -> ("error out"=w380:errorcluster)  [unwired: 8 in, 2 out]
              n192 = property on="Working..." class="Slide (strict)"("Value"=w374) -> ()  [unwired: 2 in, 2 out]
              n193 = call "Simple Wait.vi"("mS"=u32 200, "error in"=w380) -> ("error out"=w379:errorcluster)  [unwired: 12 in, 1 out]
              n194 = call <vilib>:"Simple Error Handler.vi"("error in (no error)"=w379) -> ()  [unwired: 4 in, 5 out]
            }
            frame #6 {
              n195 = Unbundle By Name(w397) -> ()  [unwired: 1 out]
              n196 = Split 1D Array(array=w396, index=64) -> (second subarray=w393:u8[])  [unwired: 1 out]
              n197 = Array Size(array=w393) -> (size(s)=w392:i32)
              n198 = while {
                shift-right: [w403] -> _
                shift-left: _ -> [_]
                shift-right: [w411] -> _
                shift-left: w393 -> [w400]
                shift-right: [w407] -> _
                shift-left: u16 16384 -> [w409]
                tunnel: w392 -> [w401]
                stop <- w408 stop-if-true
                n199 = Array Size(array=w400) -> (size(s)=w399:i32)
                n200 = Greater?(x=w399, y=u16 128) -> (0:w412:bool)
                n201 = case shown="True" w412 {
                  tunnel: w399 -> [w421 w423]
                  tunnel: [u16 0 w425] -> w403
                  tunnel: [w421 w424] -> w405
                  frame #0 {
                  }
                  frame #1 {
                    w424 = u16 128 ("y")
                    n202 = Subtract(x=w423, y=w424) -> (x-y=w425:i32)
                  }
                }
                n203 = Add(x=w405, y=w409) -> (x+y=w407:i32)
                n204 = Split 1D Array(array=w400, index=w405) -> (first subarray=w410:u8[], second subarray=w411:u8[])
                n205 = Equal To 0?(x=w403) -> (x = 0?=w408:bool)
                n206 = case shown="1, Default" w405 {
                  selector: w405 -> [_ w417]
                  tunnel: w410 -> [_ w420]
                  tunnel: w409 -> [_ w419]
                  tunnel: T3."Write Block" ("Function") -> [_ w418]
                  frame #0 {
                  }
                  frame #1 {
                    n207 = call "JTAG F-RAM.vi"("Function"=w418, "Address"=w419, "Blocksize"=w417, "Block Write Data"=w420) -> ("error out"=w415:errorcluster)  [unwired: 9 in, 2 out]
                    n208 = call "Simple Wait.vi"("mS"=u32 100, "error in"=w415) -> ("error out"=w414:errorcluster)  [unwired: 12 in, 1 out]
                    n209 = call <vilib>:"Simple Error Handler.vi"("error in (no error)"=w414) -> ()  [unwired: 4 in, 5 out]
                  }
                }
                n210 = Subtract(x=w401, y=w403) -> (x-y=w402:i32)
                n211 = Divide(x=w402, y=w401) -> (x/y=w404:dbl)
                n212 = property on="Working..." class="Slide (strict)"("Value"=w404) -> ()  [unwired: 2 in, 2 out]
              }
            }
            frame #7 {
              n213 = call "JTAG F-RAM.vi"("Function"=T3."Power DN") -> ("error out"=w426:errorcluster)  [unwired: 12 in, 2 out]
              n214 = call <vilib>:"Simple Error Handler.vi"("error in (no error)"=w426) -> ()  [unwired: 4 in, 5 out]
            }
          }
        }
      }
      frame #5 {
        w434 = u8[] []  # Data
        w435 = u16[] []  # Addresses
        n215 = local read "Front Panel"() -> (w431:T1)
        n216 = for {
          N: 5 -> [_]
          shift-right: [w437] -> _
          shift-left: w435 -> [w442]
          shift-right: [w438] -> _
          shift-left: w434 -> [w441]
          shift-right: [w436] -> w430
          shift-left: w431 -> [w439]
          i -> [w440]
          n217 = case shown="1" w440 {
            tunnel: w442 -> [_ w484 w598 w607 w624]
            tunnel: w441 -> [_ w482 w522 w601 w625]
            tunnel: w439 -> [w447 w481 w591 w605 w621]
            tunnel: [w445 w483 w522 w601 w625] -> w438
            tunnel: [w451 w485 w598 w607 w624] -> w437
            tunnel: [w447 w480 w593 w606 w621] -> w436
            frame #0 {
              w448 = u16 64 ("Blocksize")
              n218 = call "JTAG F-RAM.vi"("Function"=T3."Power UP") -> ("error out"=w450:errorcluster)  [unwired: 12 in, 2 out]
              n219 = call "JTAG F-RAM.vi"("Function"=T3."Read Block", "Address"=u16 32704, "error in (no error)"=w450, "Blocksize"=w448) -> ("Block Read Data"=w452:u16[], "error out"=w449:errorcluster)  [unwired: 9 in, 1 out]
              n220 = To Unsigned Byte Integer(number=w452) -> (unsigned 8bit integer=w445:u8[])
              n221 = call <vilib>:"Simple Error Handler.vi"("error in (no error)"=w449) -> ()  [unwired: 4 in, 5 out]
              n222 = for {
                N: w448 -> [_]
                tunnel: [w457] -> w451 mode=indexing
                i -> [w455]
                n223 = To Unsigned Word Integer(number=w455) -> (unsigned 16bit integer=w456:u16)
                n224 = Multiply(x=w456, y=u16 1) -> (x*y=w458:u16)
                n225 = Add(x=w458, y=u16 32704) -> (x+y=w457:u16)
              }
              n226 = property on="Working..." class="Slide (strict)"("Visible"=TRUE, "Value"=0.0) -> ()  [unwired: 2 in, 2 out]
            }
            frame #1 {
              w472 = u8[] []  # Data
              w479 = T3."Read Single" ("Function")
              n227 = call "JTAG F-RAM.vi"("Function"=w479, "Address"=u16 16384) -> ("Read Value"=w476:u8, "error out"=w464:errorcluster)  [unwired: 11 in, 1 out]
              n228 = call "Simple Wait.vi"("mS"=u32 40, "error in"=w464) -> ("error out"=w465:errorcluster)  [unwired: 12 in, 1 out]
              n229 = call "JTAG F-RAM.vi"("Function"=w479, "Address"=u16 16385, "error in (no error)"=w465) -> ("Read Value"=w475:u8, "error out"=w470:errorcluster)  [unwired: 10 in, 1 out]
              n230 = Join Numbers(hi=w475, lo=w476) -> ((hi.lo)=w469:u16)
              n231 = In Range and Coerce(upper limit=u16 2047, x=w469, lower limit=u16 0) -> (coerced(x)=w463:u16)  [unwired: 1 out]
              n232 = call <vilib>:"Simple Error Handler.vi"("error in (no error)"=w470) -> ()  [unwired: 4 in, 5 out]
              n233 = Multiply(x=w463, y=u16 3) -> (x*y=w461:u16)
              n234 = Bundle By Name(cluster=w481, "# of Entries"=w463) -> (w480:T1)
              n235 = while {
                shift-right: [w502] -> _
                shift-left: u16 16386 -> [w501]
                shift-right: [w495] -> _
                shift-left: w461 -> [w505]
                shift-right: [w500] -> w471
                shift-left: w472 -> [w499]
                tunnel: w461 -> [w492]
                stop <- w504 stop-if-true
                n236 = Greater?(x=w505, y=u16 128) -> (0:w506:bool)
                n237 = case shown="True" w506 {
                  tunnel: w505 -> [w516 w518]
                  tunnel: [u16 0 w520] -> w495
                  tunnel: [w516 w519] -> w498
                  frame #0 {
                  }
                  frame #1 {
                    w519 = u8 128 ("y")
                    n238 = Subtract(x=w518, y=w519) -> (x-y=w520:u16)
                  }
                }
                n239 = Add(x=w498, y=w501) -> (x+y=w502:u16)
                n240 = case shown="1, Default" w498 {
                  selector: w498 -> [_ w513]
                  tunnel: T3."Read Block" ("Function") -> [_ w515]
                  tunnel: w501 -> [_ w514]
                  tunnel: [u8[] [] w512] -> w497
                  frame #0 {
                  }
                  frame #1 {
                    n241 = call "JTAG F-RAM.vi"("Function"=w515, "Address"=w514, "Blocksize"=w513) -> ("Block Read Data"=w512:u16[], "error out"=w509:errorcluster)  [unwired: 10 in, 1 out]
                    n242 = call "Simple Wait.vi"("mS"=u32 100, "error in"=w509) -> ("error out"=w510:errorcluster)  [unwired: 12 in, 1 out]
                    n243 = call <vilib>:"Simple Error Handler.vi"("error in (no error)"=w510) -> ()  [unwired: 4 in, 5 out]
                  }
                }
                n244 = Subtract(x=w492, y=w495) -> (x-y=w493:u16)
                n245 = To Unsigned Byte Integer(number=w497) -> (unsigned 8bit integer=w496:u8[])
                n246 = Divide(x=w493, y=w492) -> (x/y=w494:dbl)
                n247 = Equal To 0?(x=w495) -> (x = 0?=w504:bool)
                n248 = property on="Working..." class="Slide (strict)"("Value"=w494) -> ()  [unwired: 2 in, 2 out]
                n249 = Build Array (concatenate)(w499, w496) -> (w500:u8[])
              }
              n250 = for {
                N: w463 -> [_]
                tunnel: [w488] -> w473 mode=indexing
                i -> [w486]
                n251 = To Unsigned Word Integer(number=w486) -> (unsigned 16bit integer=w487:u16)
                n252 = Multiply(x=w487, y=u16 1) -> (x*y=w489:u16)
                n253 = Add(x=w489, y=u16 16386) -> (x+y=w488:u16)
              }
              n254 = Build Array (concatenate)(w484, w473) -> (w485:u16[])
              n255 = Build Array (concatenate)(w482, w471) -> (w483:u8[])
            }
            frame #2 {
              w590 = 16 ("length")
              n256 = Array Subset(array=w522, index=16, length=w590) -> (w586:u8[])
              n257 = Array Subset(array=w522, index=32, length=w590) -> (w585:u8[])
              n258 = Array Subset(array=w522, index=48, length=w590) -> (w584:u8[])
              n259 = Index Array(array=w522, index=5) -> (element=w521:u8)
              n260 = Index Array(array=w522, index=0) -> (element=w582:u8)
              n261 = Index Array(array=w522, index=1) -> (element=w570:u8)
              n262 = Number To Boolean Array(number=w582) -> (Boolean array=w581:bool[])
              n263 = Number To Boolean Array(number=w570) -> (Boolean array=w569:bool[])
              n264 = Array To Cluster(array=w581) -> (cluster=w580:T7)
              n265 = Array To Cluster(array=w569) -> (cluster=w568:T7)
              n266 = Unbundle(w580) -> ("Boolean array[0]"=w579:bool, "Boolean array[1]"=w578:bool, "Boolean array[2]"=w577:bool, "Boolean array[3]"=w576:bool, "Boolean array[4]"=w575:bool, "Boolean array[5]"=w574:bool, "Boolean array[6]"=w573:bool, "Boolean array[7]"=w572:bool)
              n267 = Unbundle(w568) -> ("Boolean array[0]"=w567:bool, "Boolean array[1]"=w566:bool, "Boolean array[2]"=w565:bool, "Boolean array[3]"=w564:bool, "Boolean array[4]"=w563:bool, "Boolean array[5]"=w562:bool, "Boolean array[6]"=w561:bool, "Boolean array[7]"=w560:bool)
              n268 = Bundle By Name(cluster=w591, "PWR_TRIMS (0x7FD0-7FDF"=w586, "STIM_TRIMS (0x7FE0-7FEF"=w585, "MICS_TRIMS (0x7FF0-7FFF"=w584, "0x7FC5 - STIM ASIC REV"=w521) -> (w592:T1)
              n269 = Bundle By Name "0x7FC0 - Startup"(cluster=w592, "Set UV_PROT"=w579, "Set LDO_CTL"=w578, "Set PWR Trim Defaults"=w577, "Do STIM Digital Startup"=w576, "Do STIM BBC Startup"=w575, "Do MICS Startup"=w574, "<Reserved - $40> 5"=w573, "<Reserved - $80> 5"=w572) -> (w597:T1)
              n270 = Bundle By Name "0x7FC1 - STIM TRIMS"(cluster=w597, "Set BG_TRIM"=w567, "Set CG_TRIM"=w566, "Set PGO_TRIM"=w565, "Set CM_TRIM"=w564, "<Reserved - $10> 3"=w563, "<Reserved - $20> 3"=w562, "<Reserved - $40> 3"=w561, "<Reserved - $80> 3"=w560) -> (w596:T1)
              n271 = Index Array(array=w522, index=2) -> (element=w558:u8)
              n272 = Index Array(array=w522, index=3) -> (element=w546:u8)
              n273 = Index Array(array=w522, index=4) -> (element=w541:u8)
              n274 = Number To Boolean Array(number=w558) -> (Boolean array=w557:bool[])
              n275 = Number To Boolean Array(number=w546) -> (Boolean array=w545:bool[])
              n276 = Number To Boolean Array(number=w541) -> (Boolean array=w540:bool[])
              n277 = Array To Cluster(array=w557) -> (cluster=w556:T7)
              n278 = Array To Cluster(array=w545) -> (cluster=w544:T7)
              n279 = Array To Cluster(array=w540) -> (cluster=w539:T7)
              n280 = Unbundle(w556) -> ("Boolean array[0]"=w555:bool, "Boolean array[1]"=w554:bool, "Boolean array[2]"=w553:bool, "Boolean array[3]"=w552:bool, "Boolean array[4]"=w551:bool, "Boolean array[5]"=w550:bool, "Boolean array[6]"=w549:bool, "Boolean array[7]"=w548:bool)
              n281 = Unbundle(w544) -> ("Boolean array[0]"=w543:bool, "Boolean array[1]"=w537:bool, "Boolean array[2]"=w536:bool, "Boolean array[3]"=w535:bool, "Boolean array[4]"=w534:bool, "Boolean array[5]"=w533:bool, "Boolean array[6]"=w532:bool, "Boolean array[7]"=w531:bool)
              n282 = Unbundle(w539) -> ("Boolean array[0]"=w538:bool, "Boolean array[1]"=w530:bool, "Boolean array[2]"=w529:bool, "Boolean array[3]"=w528:bool, "Boolean array[4]"=w527:bool, "Boolean array[5]"=w526:bool, "Boolean array[6]"=w525:bool, "Boolean array[7]"=w524:bool)
              n283 = Bundle By Name "0x7FC4 - SPCL TEST"(cluster=w596, "Exec STIM Program"=w538, "MICS 400 CW XMIT"=w530, "HALT Test Sequence"=w529, "<Reserved - $08> 4"=w528, "<Reserved - $10> 4"=w527, "<Reserved - $20> 4"=w526, "<Reserved - $40> 4"=w525, "Use ePG LED's w/MP"=w524) -> (w595:T1)
              n284 = Bundle By Name "0x7FC3 - MICS TRIMS"(cluster=w595, "Apply MICS Trims"=w543, "Exec CALIBRATIONS"=w537, "<Reserved - $04>"=w536, "<Reserved - $10>"=w535, "<Reserved - $10>"=w534, "<Reserved - $20>"=w533, "<Reserved - $40>"=w532, "Apply MICS Trims"=w531) -> (w594:T1)
              n285 = Bundle By Name "0x7FC2 - PWR TRIMS"(cluster=w594, "<Reserved - $01> 2"=w555, "<Reserved - $02> 2"=w554, "<Reserved - $04> 2"=w553, "<Reserved - $08> 2"=w552, "<Reserved - $10> 2"=w551, "<Reserved - $20> 2"=w550, "<Reserved - $40> 2"=w549, "<Reserved - $80> 2"=w548) -> (w593:T1)
            }
            frame #3 {
              n286 = Unbundle By Name(w605) -> ("# of Entries"=w604:u16)
              n287 = Split 1D Array(array=w601, index=64) -> (second subarray=w600:u8[])  [unwired: 1 out]
              n288 = for {
                N: w604 -> [_]
                shift-right: [w620] -> w602
                shift-left: cluster{"Address":u16, "Data":u8}[] [] ("STIM PROGRAM FRAM DATA") -> [w619]
                shift-right: [w617] -> _
                shift-left: w600 -> [w618]
                n289 = Split 1D Array(array=w618, index=3) -> (first subarray=w613:u8[], second subarray=w617:u8[])
                n290 = Array To Cluster(array=w613) -> (cluster=w611:cluster{"[0]":u8, "[1]":u8, "[2]":u8})
                n291 = Unbundle(w611) -> ("[0]"=w610:u8, "[1]"=w609:u8, "[2]"=w608:u8)
                n292 = Join Numbers(hi=w609, lo=w610) -> ((hi.lo)=w612:u16)
                n293 = Bundle By Name(cluster=cluster{"Address":u16, "Data":u8} {"Address"=0, "Data"=0} ("Cluster"), "Address"=w612, "Data"=w608) -> (w614:cluster{"Address":u16, "Data":u8})
                n294 = Build Array (concatenate)(w619, w614) -> (w620:cluster{"Address":u16, "Data":u8}[])
              }
              n295 = Bundle By Name(cluster=w605, "FRAM STIM DATA"=w602) -> (w606:T1)
            }
            frame #4 {
              n296 = call "JTAG F-RAM.vi"("Function"=T3."Power DN") -> ("error out"=w622:errorcluster)  [unwired: 12 in, 2 out]
              n297 = call <vilib>:"Simple Error Handler.vi"("error in (no error)"=w622) -> ()  [unwired: 4 in, 5 out]
            }
          }
        }
        n298 = local write "Front Panel"(w430) -> ()
      }
    }
    n299 = local read "Front Panel"() -> (w7:T1)
    n300 = Unbundle By Name(w7) -> ("User Controls.Exit"=w6:bool)
  }
  n301 = stacked-sequence {
    tunnel: w3 -> [_]
    frame #0 {
      w629 = FALSE ("User Controls.Read from F-Ram")
      n302 = property on="Working..." class="Slide (strict)"("Visible"=FALSE) -> ()  [unwired: 2 in, 2 out]
      n303 = local read "Front Panel"() -> (w628:T1)
      n304 = Bundle By Name(cluster=w628, "User Controls.Read from F-Ram"=w629, "User Controls.Write to F-Ram"=w629, "User Controls.Import Stim Prog"=w629, "User Controls.Exit"=w629) -> (w627:T1)
      n305 = local write "Front Panel"(w627) -> ()
    }
  }
